vi "Configure Channel Characteristics.vi"(4 "Invert (F: False)":bool, 6 "Vernier (F: False)":bool, 7 "Input Impedance (1: 1 Mohms)":i16(ring)=1 items=["50 ohms", "1 Mohms"], 8 "error in (no error)":errorcluster, 9 "BW Limit (F: False)":bool, 10 "Channel (0: Channel 1)":u16(ring) items=["Channel 1", "Channel 2", "Channel 3", "Channel 4"], 11 "VISA resource name":refnum<visa-resource-name>) -> (0 "error out":errorcluster, 3 "VISA resource name out":refnum<visa-resource-name>)   [LabVIEW 2017, in "Agilent 6000 Series.lvlib"]
doc: "This VI configures the attributes that control the electrical characteristics of the channel. These properties are the input impedance, bandwidth limit, vernier and invert."
uses:
  <instrlib>/Agilent 6000 Series/Agilent 6000 Series.lvlib
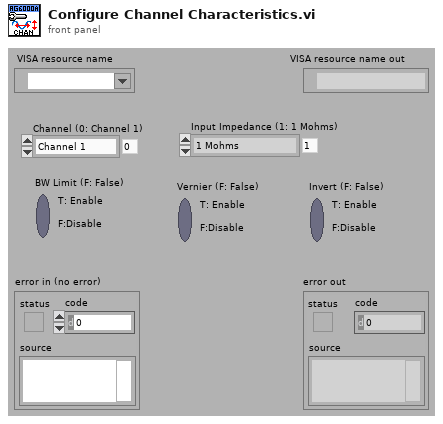
[diagram p1: front panel]
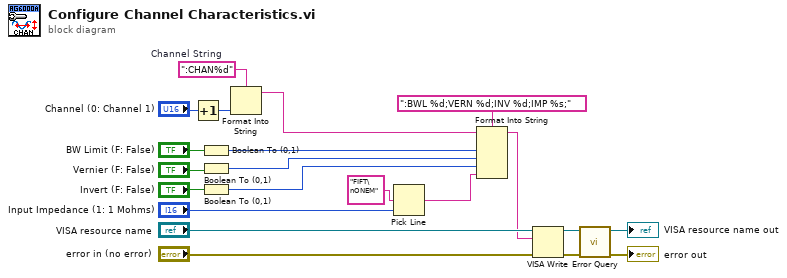
[diagram p0: block diagram]
diagram:
  w15 = ":CHAN%d"  # Channel String
  n1 = Increment(x="Channel (0: Channel 1)") -> (x+1=w1:u16)
  n2 = Boolean To (0,1)(Boolean="BW Limit (F: False)") -> (0, 1=w10:i16)
  n3 = Boolean To (0,1)(Boolean="Vernier (F: False)") -> (0, 1=w5:i16)
  n4 = Boolean To (0,1)(Boolean="Invert (F: False)") -> (0, 1=w4:i16)
  n5 = Format Into String(format string=w15, w1) -> (resulting string=w6:string)  [unwired: 2 in, 1 out]
  n6 = Pick Line(multi-line string="FIFT\nONEM" ("string (\"\")"), line index="Input Impedance (1: 1 Mohms)") -> (output string=w3:string)  [unwired: 1 in]
  n7 = Format Into String(format string=":BWL %d;VERN %d;INV %d;IMP %s;", initial string=w6, w10, w5, w4, w3) -> (resulting string=w8:string)  [unwired: 1 in, 1 out]
  n8 = VISA Write(VISA resource name="VISA resource name", write buffer=w8, error in (no error)="error in (no error)") -> (VISA resource name out=w17:refnum<visa-resource-name>, error out=w16:errorcluster)  [unwired: 1 out]
  n9 = call <instrlib>:"Error Query.vi"("error in (no error)"=w16, "VISA resource name"=w17) -> ("error out"=→"error out":errorcluster, "VISA resource name out"=→"VISA resource name out":refnum<visa-resource-name>)  [unwired: 6 in, 2 out]
